vi "write&read.vi"(8 "错误输入（无错误）":errorcluster, 10 "Write Buffer":string="SENS:DATA?" caption="写入缓冲区", 11 "VISA GPIB Resource":refnum<visa-resource-name>="GPIB0::2::INSTR" caption="VISA GPIB资源") -> (0 "错误输出":errorcluster, 2 "Read Buffer":string caption="读取缓冲区", 3 "VISA资源名称输出":refnum<visa-resource-name>)   [LabVIEW 2017]
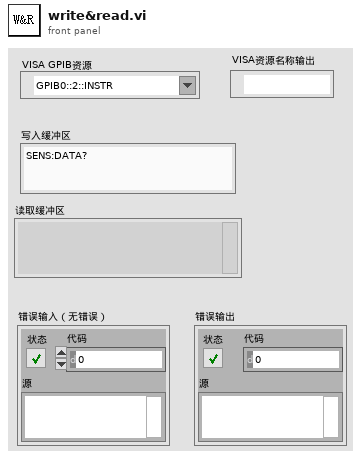
[diagram p1: front panel]
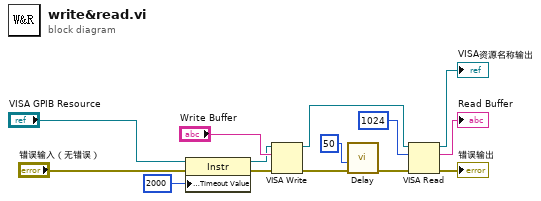
[diagram p0: block diagram]
diagram:
  n1 = property class="Instr"(reference="VISA GPIB Resource", error in="错误输入（无错误）", "General Settings:Timeout Value"=u32 2000) -> (reference out=w11:refnum<visa-resource-name>, error out=w10:errorcluster)
  n2 = VISA Write(VISA resource name=w11, write buffer="Write Buffer", error in (no error)=w10) -> (VISA resource name out=w9:refnum<visa-resource-name>, error out=w2:errorcluster)  [unwired: 1 out]
  n3 = call "Delay.vi"("error in (no error)"=w2, "Delay"=u32 50 ("milliseconds to wait")) -> ("error out"=w3:errorcluster)  [unwired: 9 in]
  n4 = VISA Read(VISA resource name=w9, byte count=u32 1024 ("字节总数"), error in (no error)=w3) -> (VISA resource name out=→"VISA资源名称输出":refnum<visa-resource-name>, read buffer=→"Read Buffer":string, error out=→"错误输出":errorcluster)  [unwired: 1 out]
